vi "updateILCOutputs.vi"(8 "error in (no error)":errorcluster, 11 "Model in":refnum<class "Model.lvclass">) -> (0 "error out":errorcluster, 3 "Model out":refnum<class "Model.lvclass">)   [LabVIEW 2013, in "Model.lvclass"]
uses:
  Model.lvclass
  <userlib>/Common/ILC/Typedefs/OutputData.ctl
  Model.lvclass/Model.ctl
  <userlib>/Common/Devices/StepperMotor/StepperMotor/StepperMotor.lvclass/StepperMotor.ctl
  <userlib>/Common/ILC/ILC/ILC.lvclass/ILC.ctl
  <userlib>/Common/ILC/ILC/ILC.lvclass
  <userlib>/Common/ILC/Typedefs/ILCTypedefs.lvlib
  <userlib>/Common/Devices/StepperMotor/StepperMotor/StepperMotor.lvclass
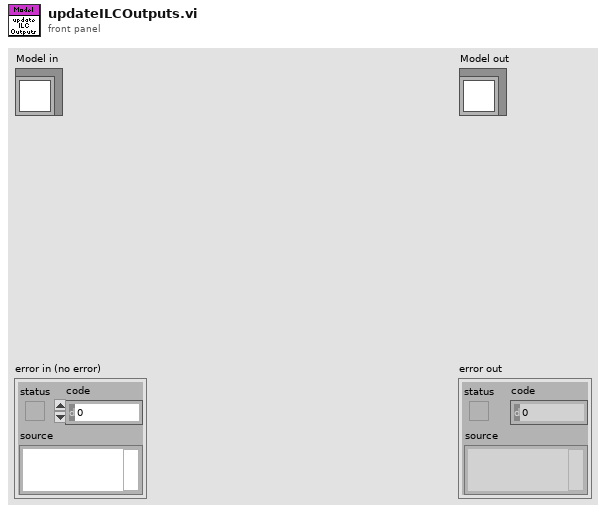
[diagram p1: front panel]
types:
  T1 = typedef "ILCCommon.lvlib/ILCTypedefs.lvlib/OutputData.ctl" = cluster{"Step & Direction":i16, "Blower RPM":u8, "PWM (SSR)":u8, "Ch1":u16, "Ch2":u16, "Ch3":u16, "Ch4":u16}
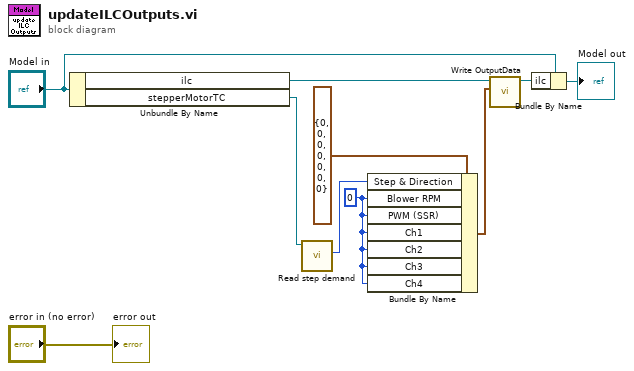
[diagram p0: block diagram]
diagram:
  w4 = u8 0 ("Blower RPM")
  n1 = Unbundle By Name("Model in") -> ("ilc"=w8:refnum<class "ILC.lvclass">, "stepperMotorTC"=w6:refnum<class "StepperMotorTC.lvclass">)
  n2 = call <userlib>:"Read step demand.vi"("StepperMotor in"=w6) -> ("step demand"=w5:i16)  [unwired: 9 in, 1 out]
  n3 = Bundle By Name(cluster=T1 {"Step & Direction"=0, "Blower RPM"=0, "PWM (SSR)"=0, "Ch1"=0, "Ch2"=0, "Ch3"=0, "Ch4"=0} ("OutputData"), "Step & Direction"=w5, "Blower RPM"=w4, "PWM (SSR)"=w4, "Ch1"=w4, "Ch2"=w4, "Ch3"=w4, "Ch4"=w4) -> (w1:T1)
  n4 = call <userlib>:"Write OutputData.vi"("OutputData"=w1, "ILC in"=w8) -> ("ILC out"=w2:refnum<class "ILC.lvclass">)  [unwired: 9 in]
  n5 = Bundle By Name(cluster="Model in", "ilc"=w2) -> (→"Model out":refnum<class "Model.lvclass">)
  "error out" <- "error in (no error)"
